vi "State Order.vi"(8 "Fehler (Eingang)":errorcluster, 11 "Options":T2) -> (0 "Fehler (Ausgang)":errorcluster, 3 "States":T1[](array[typedef]))   [LabVIEW 2014]
doc: "Dieses VI erstellt basierend auf dem Eingang \"Waschprogramme\" ein Array aus Zuständen, die für die entsprechenden Waschprogramme ausgeführt werden."
uses:
  Controls/Wash Options.ctl
  Controls/State Control Enum.ctl
panel:
  # "Eingänge"
  # "Ausgänge"
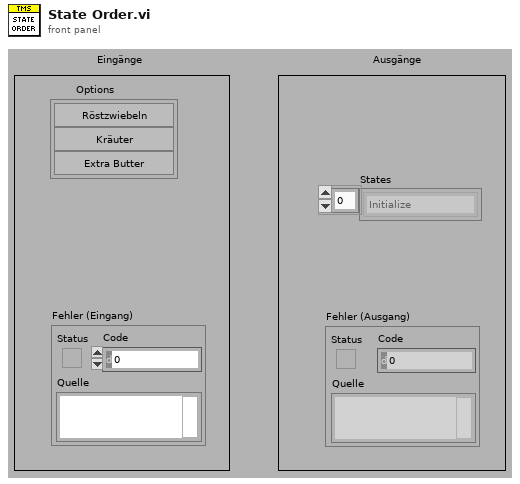
[diagram p1: front panel]
types:
  T1 = typedef "State Control Enum.ctl" = enum16{"Initialize", "Wait for Start", "Plate Dispension", "Spätzle Dispension", "Heating", "Cheese Dispension", "Onion Dispension", "Garlic Dispension", "Butter Dispension", "Move to Spätzle", "Move To Cheese", "Move to Exit", "Stop", "Skip"}
  T2 = typedef "Wash Options.ctl" = cluster{"Röstzwiebeln":bool, "Kräuter":bool, "Extra Butter":bool}
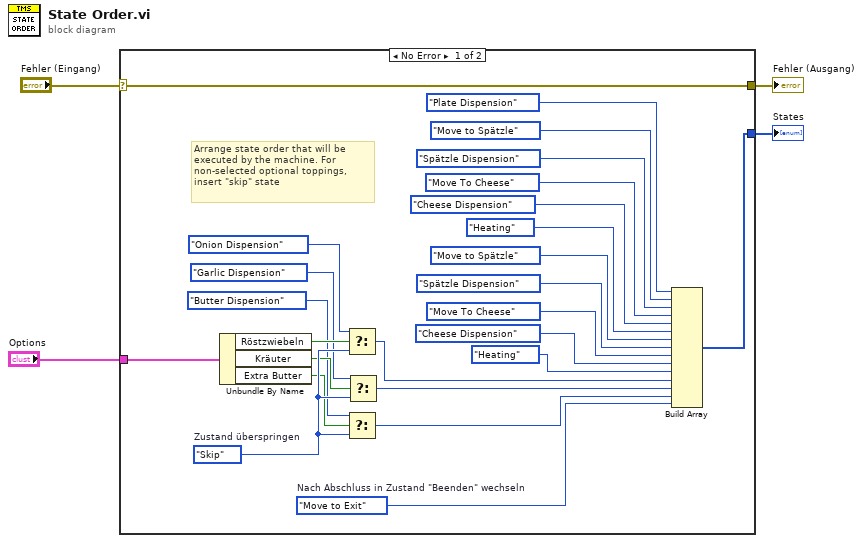
[diagram p0: block diagram]
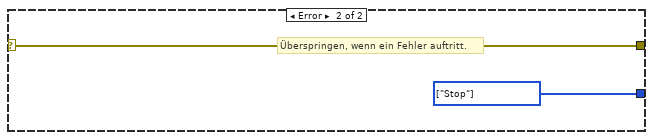
[diagram p2: hidden frame]
diagram:
  n1 = case "Case-Struktur" shown="No Error" "Fehler (Eingang)" {
    selector: "Fehler (Eingang)" -> [w8 w31]
    tunnel: "Options" -> [w24 _]
    tunnel: [w7 w30] -> w3
    tunnel: [w8 w31] -> w1
    frame No Error {
      w29 = State_Control_Enum."Move to Exit"  # Nach Abschluss in Zustand "Beenden" wechseln
      w28 = State_Control_Enum."Skip"  # Zustand überspringen
      # "Arrange state order that will be executed by the machine. For non-selected optional toppings,\ninsert \"skip\" state"
      n2 = Unbundle By Name ("Nach Namen aufschlüsseln")(w24) -> ("Röstzwiebeln"=w23:bool, "Kräuter"=w22:bool, "Extra Butter"=w21:bool)
      n3 = Select ("Auswählen")(t=State_Control_Enum."Onion Dispension" ("Zustandselement"), s=w23, f=w28) -> (s? t:f=w25:T1)
      n4 = Select ("Auswählen")(t=State_Control_Enum."Butter Dispension" ("Zustandselement"), s=w21, f=w28) -> (s? t:f=w27:T1)
      n5 = Select ("Auswählen")(t=State_Control_Enum."Garlic Dispension" ("Zustandselement"), s=w22, f=w28) -> (s? t:f=w26:T1)
      n6 = Build Array ("Array erstellen")(State_Control_Enum."Plate Dispension" ("Zustandselement"), State_Control_Enum."Move to Spätzle" ("Trocknen"), State_Control_Enum."Spätzle Dispension" ("Zustandselement"), State_Control_Enum."Move To Cheese" ("Zustandselement"), State_Control_Enum."Cheese Dispension" ("Zustandselement"), State_Control_Enum."Heating" ("Zustandselement"), State_Control_Enum."Move to Spätzle" ("Trocknen"), State_Control_Enum."Spätzle Dispension" ("Zustandselement"), State_Control_Enum."Move To Cheese" ("Zustandselement"), State_Control_Enum."Cheese Dispension" ("Zustandselement"), State_Control_Enum."Heating" ("Zustandselement"), w25, w26, w27, w29) -> (w7:T1[])
    }
    frame Error {
      w30 = T1[] [enum."Stop"] items=["Initialize", "Wait for Start", "Plate Dispension", "Spätzle Dispension", "Heating", "Cheese Dispension", "Onion Dispension", "Garlic Dispension", "Butter Dispension", "Move to Spätzle", "Move To Cheese", "Move to Exit", "Stop", "Skip"]
      # "Überspringen, wenn ein Fehler auftritt."
    }
  }
  "States" <- w3
  "Fehler (Ausgang)" <- w1
